vi "test.vi"   [LabVIEW 2014]
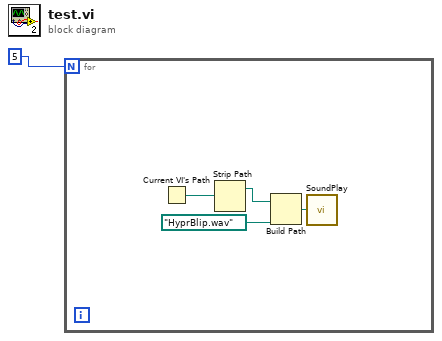
[diagram p0: block diagram]
diagram:
  n1 = for {
    N: 5 -> [_]
    n2 = Current VI's Path() -> (path=w3:path)
    n3 = Strip Path(path=w3) -> (stripped path=w2:path)  [unwired: 1 out]
    n4 = Build Path(base path=w2, name or relative path=path "HyprBlip.wav") -> (appended path=w5:path)
    n5 = call "SoundPlay.vi"("Path to Sound file"=w5) -> ()  [unwired: 2 in, 1 out]
  }
